vi "Unsubscribe from Events.vi"(8 "error in (no error)":errorcluster, 11 "Event Viewer Module in":refnum<class "Event Viewer Module.lvclass">) -> (0 "error out":errorcluster, 3 "Event Viewer Module out":refnum<class "Event Viewer Module.lvclass">)   [LabVIEW 2020, in "VolatusGUI.lvlib" / "Event Viewer Module.lvclass"]
uses:
  Event Viewer Module.lvclass
  Event Viewer Module.lvclass/Event Viewer Module.ctl
  Volatus/MessageQ/MessageQ.lvclass
  Volatus/Module/Module.lvclass
  C:/dev/lv20CE/relink/lv-volatus/Volatus/Module/Module.lvclass
  C:/dev/lv20CE/relink/lv-volatus/VolatusGUI/Event Viewer Module/Event Viewer Module.lvclass
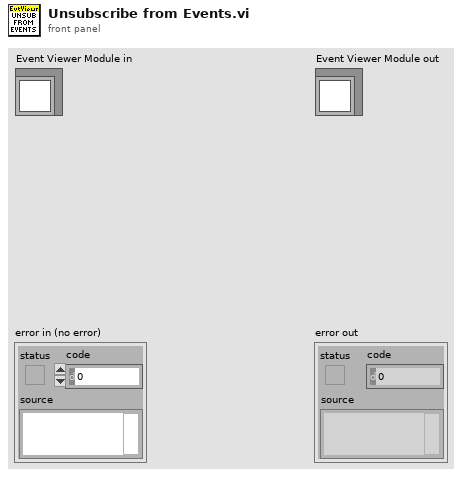
[diagram p1: front panel]
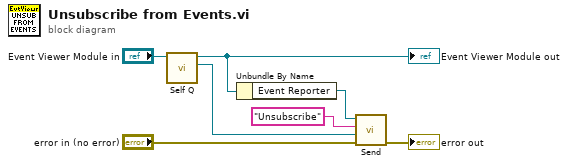
[diagram p0: block diagram]
diagram:
  n1 = call "Self Q.vi"("Module in"="Event Viewer Module in") -> ("Self Q"=w4:refnum<class "MessageQ.lvclass">, "Module out"=w5:refnum<class "Event Viewer Module.lvclass">)  [unwired: 9 in]
  "Event Viewer Module out" <- w5
  n2 = Unbundle By Name(w5) -> ("Event Reporter"=w6:refnum<class "MessageQ.lvclass">)
  n3 = call "Send.vi"("error in (no error)"="error in (no error)", "Data"=w4, "ID"="Unsubscribe", "MessageQ in"=w6) -> ("error out"=→"error out":errorcluster)  [unwired: 6 in, 1 out]
